vi "draw_overlay.vi"(6 "frame index":i32, 8 "error in (no error)":errorcluster, 9 "reference stack":refnum<class "ImageCollection.lvclass">, 10 "line sections":T1(array[cluster]), 11 "PositionSignals in":refnum<class "PositionSignals.lvclass">) -> (0 "error out":errorcluster, 3 "PositionSignals out":refnum<class "PositionSignals.lvclass">)   [LabVIEW 2010, in "PositionSignals.lvclass"]
uses:
  PositionSignals.lvclass
  common/classes/ImageCollection/ImageCollection/ImageCollection.lvclass
  common/classes/Image/Image/Image.lvclass
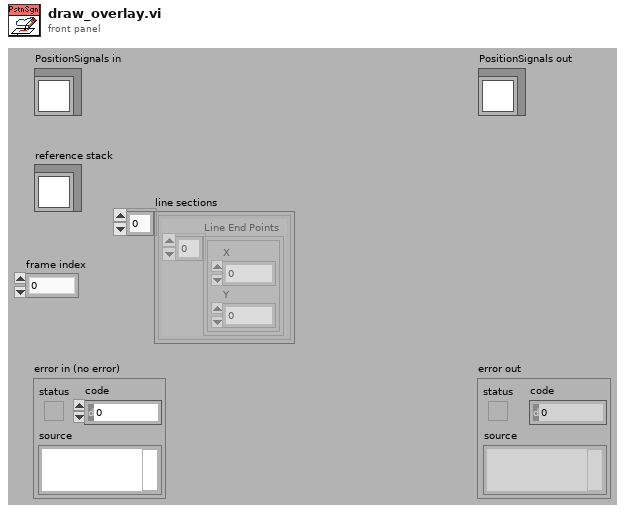
[diagram p1: front panel]
types:
  T1 = cluster{"Line End Points":cluster{"X":dbl, "Y":dbl}[]}[]
  T2 = typedef "IMAQ Image.ctl" = refnum<image>
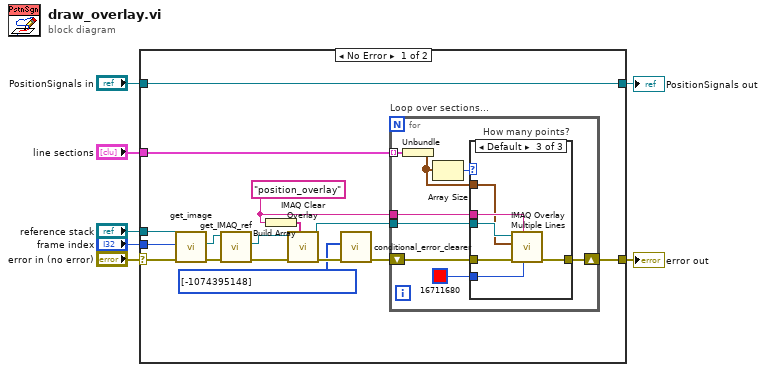
[diagram p0: block diagram]
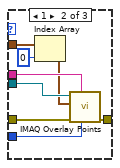
[diagram p3: hidden frame]
diagram:
  n1 = case shown="No Error" "error in (no error)" {
    selector: "error in (no error)" -> [w12 w48]
    tunnel: [w11 w48] -> w6
    tunnel: [w23 w47] -> w4
    tunnel: "PositionSignals in" -> [w23 w47]
    tunnel: "reference stack" -> [w10 _]
    tunnel: "frame index" -> [w9 _]
    tunnel: "line sections" -> [w8 _]
    frame No Error {
      w18 = "position_overlay"
      n2 = call-dynamic "get_image.vi"("error in (no error)"=w12, "index"=w9, "ImageCollection in"=w10) -> ("error out"=w22:errorcluster, "Image.lvclass"=w20:refnum<class "Image.lvclass">)  [unwired: 6 in, 1 out]
      n3 = call-dynamic "get_IMAQ_ref.vi"("error in (no error)"=w22, "Image.lvclass in"=w20) -> ("error out"=w21:errorcluster, "Image"=w19:T2)  [unwired: 5 in, 3 out]
      n4 = Build Array(w18) -> (w16:string[])
      n5 = call "IMAQ Clear Overlay"("Groups"=w16, "error in (no error)"=w21, "Image"=w19) -> ("error out"=w15:errorcluster, "Image Out"=w17:T2)  [unwired: 7 in]
      n6 = call "conditional_error_clearer.vi"("error in (no error)"=w15, "array of clearable error codes"=i32[] [-1074395148]) -> ("error out"=w14:errorcluster)  [unwired: 9 in]
      n7 = for "Loop over sections..." {
        tunnel: w17 -> [w30]
        shift-right: [w24] -> w11
        shift-left: w14 -> [w31]
        tunnel: w18 -> [w29]
        tunnel: w8 -> [w28] mode=indexing
        n8 = Unbundle(w28) -> ("Line End Points"=w27:cluster{"X":dbl, "Y":dbl}[])
        n9 = Array Size(array=w27) -> (size(s)=w26:i32)
        n10 = case "How many points?" shown="Default" w26 {
          tunnel: w31 -> [w32 w40 w45]
          tunnel: w30 -> [_ w38 w44]
          tunnel: w29 -> [_ w37 w43]
          tunnel: w27 -> [_ w35 w42]
          tunnel: u32 16711680 ("Color") -> [_ w36 w41]
          tunnel: [w32 w39 w46] -> w24
          frame 0 {
          }
          frame 1 {
            n11 = Index Array(array=w35, index=0) -> (element=w33:cluster{"X":dbl, "Y":dbl})
            n12 = call "IMAQ Overlay Points"("Color"=w36, "Group"=w37, "error in (no error)"=w40, "Point"=w33, "Image"=w38) -> ("error out"=w39:errorcluster)  [unwired: 5 in, 1 out]
          }
          frame Default {
            n13 = call "IMAQ Overlay Multiple Lines"("Color"=w41, "Group"=w43, "error in (no error)"=w45, "Line End Points"=w42, "Image"=w44) -> ("error out"=w46:errorcluster)  [unwired: 5 in, 1 out]
          }
        }
      }
    }
    frame Error {
    }
  }
  "error out" <- w6
  "PositionSignals out" <- w4
